vi "PI.vi"(2 "dt":dbl, 3 "stop_int":bool, 4 "error in (no error)":errorcluster, 5 "k_p":dbl, 6 "w_I":dbl, 7 "e":dbl) -> (0 "error out":errorcluster, 1 "u":dbl)   [LabVIEW 2019]
uses:
  discrete_control_memory.vi
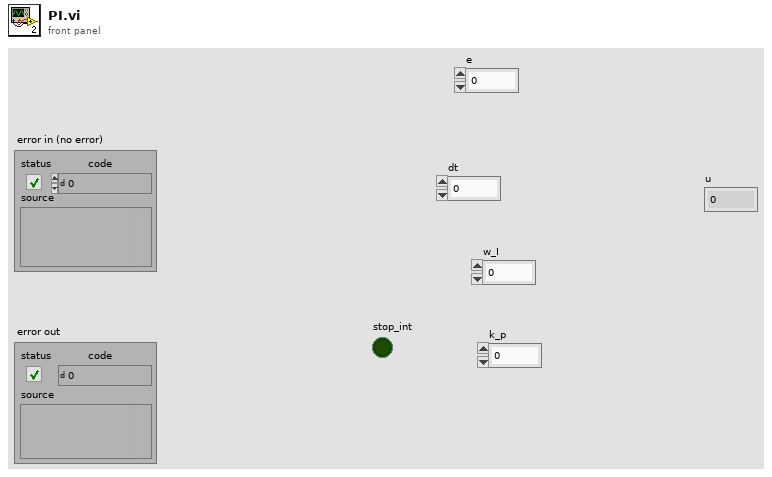
[diagram p1: front panel]
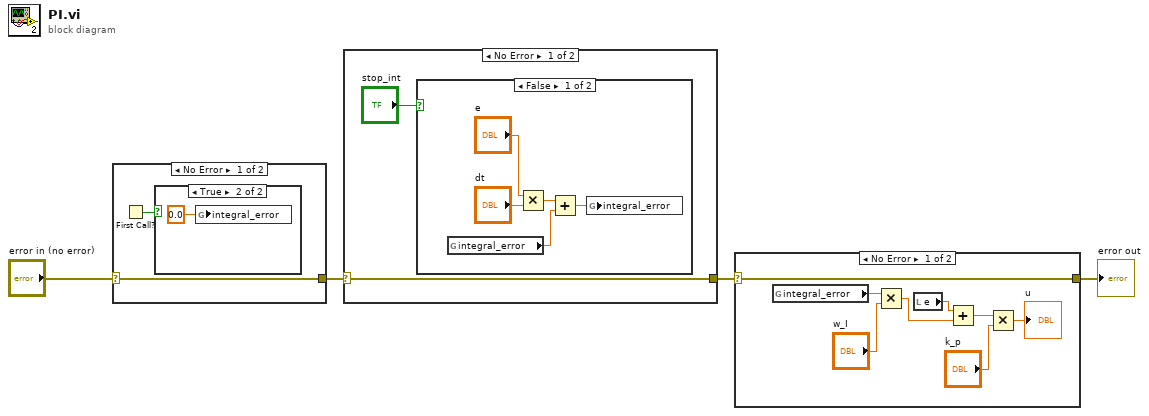
[diagram p0: block diagram]
diagram:
  n1 = case shown="No Error" "error in (no error)" {
    selector: "error in (no error)" -> [w5 w8]
    tunnel: [w5 w8] -> w3
    frame No Error {
      n2 = First Call?() -> (First Call?: T/F=w6:bool)
      n3 = case shown="True" w6 {
        frame False {
        }
        frame True {
          n4 = global write "discrete_control_memory.vi" "integral_error"(0.0 ("integral_error")) -> ()
        }
      }
    }
    frame Error {
    }
  }
  n5 = case shown="No Error" w3 {
    selector: w3 -> [w9 w16]
    tunnel: [w9 w16] -> w2
    frame No Error {
      n6 = case shown="False" "stop_int" {
        frame False {
          n7 = global read "discrete_control_memory.vi" "integral_error"() -> (w11:dbl)
          n8 = Multiply(x="e", y="dt") -> (x*y=w13:dbl)
          n9 = Add(x=w13, y=w11) -> (x+y=w12:dbl)
          n10 = global write "discrete_control_memory.vi" "integral_error"(w12) -> ()
        }
        frame True {
        }
      }
    }
    frame Error {
    }
  }
  n11 = case shown="No Error" w2 {
    selector: w2 -> [w17 w25]
    tunnel: [w17 w25] -> w1
    frame No Error {
      n12 = global read "discrete_control_memory.vi" "integral_error"() -> (w24:dbl)
      n13 = Multiply(x=w24, y="w_I") -> (x*y=w22:dbl)
      n14 = local read "e"() -> (w21:dbl)
      n15 = Add(x=w21, y=w22) -> (x+y=w20:dbl)
      n16 = Multiply(x=w20, y="k_p") -> (x*y=→"u":dbl)
    }
    frame Error {
    }
  }
  "error out" <- w1
